vi "TSM Relay Get Session Data.vi"(8 "error in":errorcluster, 10 "Pins":string[](array[string]), 11 "TSM context":T1) -> (0 "error out":errorcluster, 1 "Channel Group Ids":string[](array[string]), 2 "Channel Lists":string[](array[string]), 3 "Instrument Sessions":refnum<k15>[](array[refnum]), 5 "Pin Query Context":refnum<class "MultiplePinMultipleSessionQueryContext.lvclass">)   [LabVIEW 2019]
doc: "Returns the NI-Switch instrument sessions and channel lists required to access the pins."
uses:
  <vilib>/NI_TestStand_SemiconductorModule/NI_TestStand_Semiconductor_Module.lvlibp/PinMap/General/SemiconductorModuleContext.ctl
  <vilib>/NI_TestStand_SemiconductorModule/NI_TestStand_Semiconductor_Module.lvlibp/PinMap/PinQueryContext/MultiplePinMultipleSessionQueryContext/MultiplePinMultipleSessionQueryContext.lvclass
  <vilib>/NI_TestStand_SemiconductorModule/NI_TestStand_Semiconductor_Module.lvlibp/PinMap/Advanced/Custom Instruments/GetSessionData.vi
  <vilib>/NI_TestStand_SemiconductorModule/NI_TestStand_Semiconductor_Module.lvlibp
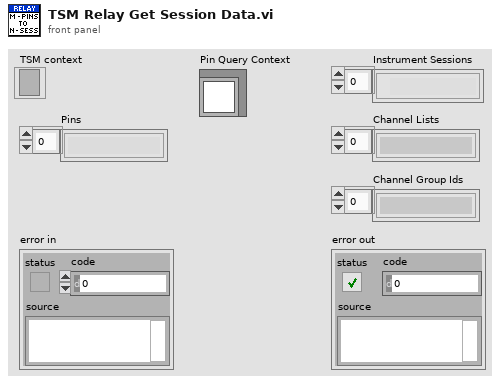
[diagram p1: front panel]
types:
  T1 = typedef "NI_TestStand_Semiconductor_Module.lvlibp/SemiconductorModuleContext.ctl" = refnum<k7>
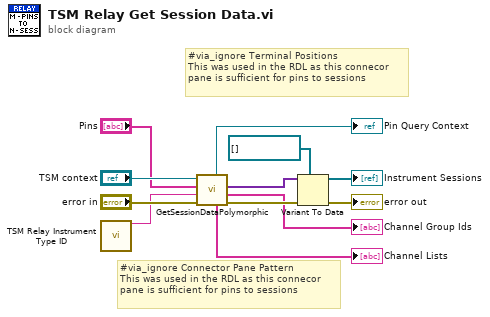
[diagram p0: block diagram]
diagram:
  # "#via_ignore Terminal Positions\nThis was used in the RDL as this connecor\npane is sufficient for pins to sessions"
  # "#via_ignore Connector Pane Pattern\nThis was used in the RDL as this connecor\npane is sufficient for pins to sessions"
  n1 = call "TSM Relay Instrument Type ID.vi"() -> ("Instrument Type ID"=w1:string)  [unwired: 15 in]
  n2 = call-poly <vilib>:"GetSessionDataPolymorphic.vi"("error in (no error)"="error in", "Instrument Type Id"=w1, "Pins"="Pins", "Semiconductor Module Context"="TSM context") -> ("error out"=w12:errorcluster, "Channel Group Ids"=→"Channel Group Ids":string[], "Session Data"=w11:variant[], "Channel Lists"=→"Channel Lists":string[], "Pin Query Context"=→"Pin Query Context":refnum<class "MultiplePinMultipleSessionQueryContext.lvclass">)  [unwired: 2 in, 1 out]
  n3 = Variant To Data(error in=w12, type=refnum<k15>[] [], Variant=w11) -> (data=→"Instrument Sessions":refnum<k15>[], error out=→"error out":errorcluster)
